vi "Special_Processing.vi"(6 "cluster in":T1, 8 "error in (no error)":errorcluster, 9 "Terminal Map In":map{string, T3}(c390), 10 "Wires":T2[](array[typedef]), 11 "GrowableObjectFunction in":refnum<class "PropertyNode.lvclass">) -> (0 "error out":errorcluster, 1 "Terminal Map Out":map{string, T3}(c390), 2 "Wires out":T2[](array[typedef]), 3 "GrowableObjectFunction out":refnum<class "PropertyNode.lvclass">)   [LabVIEW 2025, in "PropertyNode.lvclass"]
uses:
  PropertyNode.lvclass
  C:/Users/mrjak/Documents/GitHub/LVGPT/LabVIEW/VIs/Classes/Node/Node.lvclass
  Controls/wire.ctl
  Controls/Terminal.ctl
  Controls/bd.ctl
  Node.lvclass
  Node.lvclass/Node.ctl
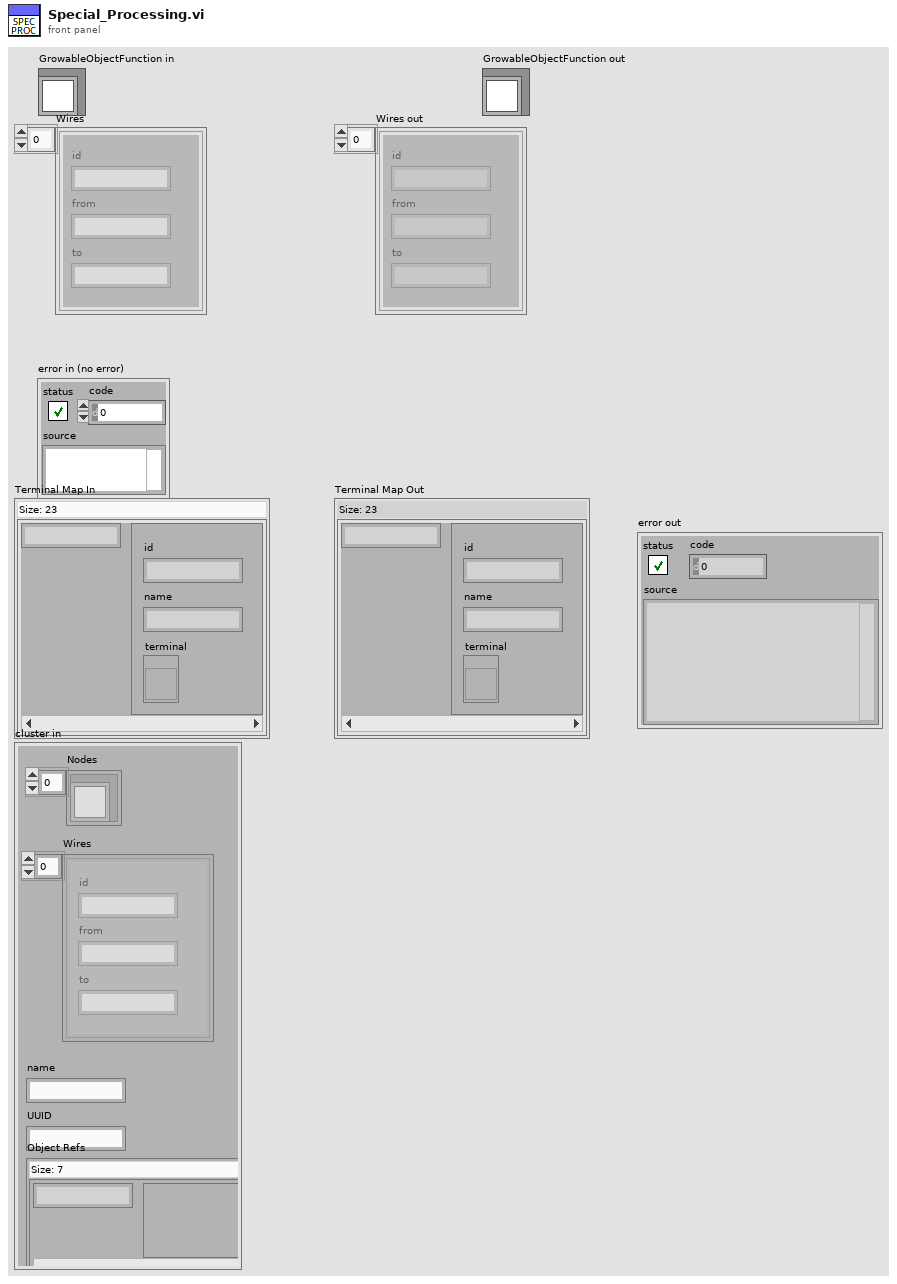
[diagram p1: front panel]
types:
  T1 = typedef "bd.ctl" = cluster{"Nodes":refnum<class "Node.lvclass">[], "Wires":T2[], "name":string, "UUID":string, "Object Refs":map{string, variant}}
  T2 = typedef "wire.ctl" = cluster{"id":string, "from":string, "to":string}
  T3 = typedef "Terminal.ctl" = cluster{"id":string, "name":string, "terminal":refnum<vi>}
  T4 = typedef "GrowableFunctionNode.ctl" = cluster{"terminalUUID":string, "Write":bool}
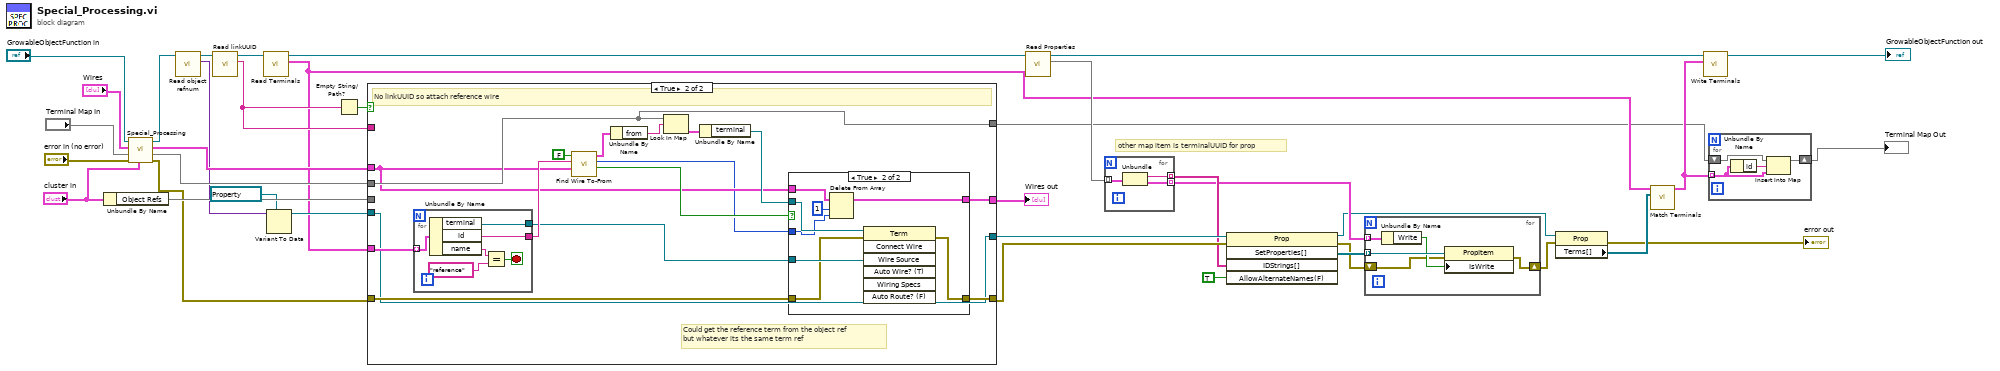
[diagram p0: block diagram]
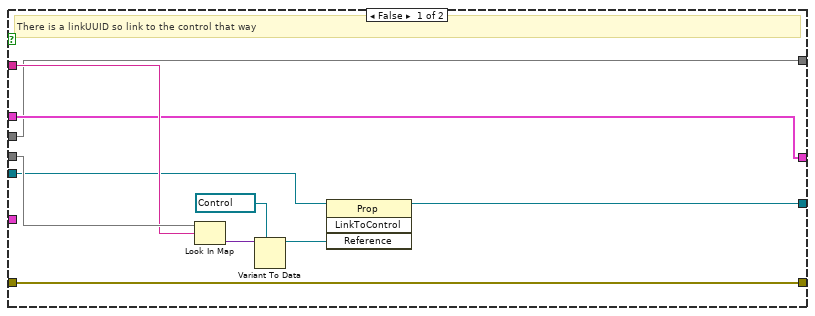
[diagram p2: hidden frame]
diagram:
  # "other map item is terminalUUID for prop"
  n1 = Unbundle By Name("cluster in") -> ("Object Refs"=w29:map{string, variant})
  n2 = call-parent "Special_Processing.vi"("cluster in"="cluster in", "error in (no error)"="error in (no error)", "Terminal Map In"="Terminal Map In", "Wires"="Wires", "Node in"="GrowableObjectFunction in") -> ("error out"=w22:errorcluster, "Terminal Map Out"=w23:map{string, T3}, "Wires out"=w26:T2[], "Node out"=w37:refnum<class "PropertyNode.lvclass">)  [unwired: 3 in]
  n3 = call-dynamic "Read object refnum.vi"("Node in"=w37) -> ("object refnum"=w18:variant, "Node out"=w32:refnum<class "PropertyNode.lvclass">)  [unwired: 8 in, 1 out]
  n4 = call-dynamic "Read linkUUID.vi"("GrowableObjectFunction in"=w32) -> ("linkUUID"=w28:string, "GrowableObjectFunction out"=w31:refnum<class "PropertyNode.lvclass">)  [unwired: 8 in, 1 out]
  n5 = call "Read Terminals.vi"("Node in"=w31) -> ("Terminals"=w12:T3[], "Node out"=w25:refnum<class "PropertyNode.lvclass">)  [unwired: 8 in, 1 out]
  n6 = Variant To Data(type=refnum<vi> refnum ("reference"), Variant=w18) -> (data=w19:refnum<vi>)  [unwired: 1 in, 1 out]
  n7 = Empty String/Path?(string/path=w28) -> (empty?=w30:bool)
  n8 = case shown="True" w30 {
    tunnel: w29 -> [w47 _]
    tunnel: w28 -> [w46 _]
    tunnel: w26 -> [w42 w50]
    tunnel: w12 -> [_ w63]
    tunnel: [w42 w48] -> w24
    tunnel: w23 -> [w40 w53]
    tunnel: w22 -> [w41 w55]
    tunnel: [w41 w54] -> w16
    tunnel: [w40 w53] -> w7
    tunnel: w19 -> [w39 w52]
    tunnel: [w38 w52] -> w17
    frame False {
      # "There is a linkUUID so link to the control that way"
      n9 = Look In Map(map=w47, key=w46) -> (value=w45:variant)  [unwired: 1 in, 1 out]
      n10 = Variant To Data(type=refnum<vi> refnum ("Reference"), Variant=w45) -> (data=w43:refnum<vi>)  [unwired: 1 in, 1 out]
      n11 = invoke class="Prop" method="LinkToControl"(reference=w39, "Reference"=w43) -> (reference out=w38:refnum<vi>)  [unwired: 2 in, 3 out]
    }
    frame True {
      # "Could get the reference term from the object ref \nbut whatever its the same term ref"
      # "No linkUUID so attach reference wire"
      n12 = for {
        tunnel: w63 -> [w79] mode=indexing
        tunnel: [w75] -> w62
        tunnel: [w74] -> w56
        stop <- w76 stop-if-true
        n13 = Unbundle By Name(w79) -> ("terminal"=w74:refnum<vi>, "id"=w75:string, "name"=w78:string)
        n14 = Equal?(x=w78, y="reference") -> (x = y?=w76:bool)
      }
      n15 = call "Find Wire To-From.vi"("Wires"=w50, "termUUID"=w62, "From UUID?"=FALSE) -> ("Found"=w51:bool, "Index"=w49:i32, "Wire"=w60:T2)  [unwired: 6 in]
      n16 = Unbundle By Name(w60) -> ("from"=w59:string)
      n17 = Look In Map(map=w53, key=w59) -> (value=w58:T3)  [unwired: 1 in, 1 out]
      n18 = Unbundle By Name(w58) -> ("terminal"=w57:refnum<vi>)
      n19 = case shown="True" w51 {
        tunnel: w57 -> [_ w73]
        tunnel: w56 -> [_ w72]
        tunnel: w55 -> [w65 w71]
        tunnel: [w65 w70] -> w54
        tunnel: w50 -> [w64 w69]
        tunnel: w49 -> [_ w67]
        tunnel: [w64 w66] -> w48
        frame False {
        }
        frame True {
          n20 = Delete From Array(array=w69, length=1, index=w67) -> (array with subset deleted=w66:T2[])  [unwired: 1 out]
          n21 = invoke class="Term" method="Connect Wire"(reference=w73, error in=w71, "Wire Source"=w72) -> (error out=w70:errorcluster)  [unwired: 4 in, 6 out]
        }
      }
    }
  }
  "Wires out" <- w24
  n22 = call-dynamic "Read Properties.vi"("PropertyNode in"=w25) -> ("Properties"=w15:map{string, T4}, "PropertyNode out"=w21:refnum<class "PropertyNode.lvclass">)  [unwired: 8 in, 1 out]
  n23 = for {
    tunnel: w15 -> [w82] mode=indexing
    tunnel: [w81] -> w14 mode=indexing
    tunnel: [w80] -> w4 mode=indexing
    n24 = Unbundle(w82) -> (w81:string, "GrowableFunctionNode"=w80:T4)
  }
  n25 = invoke class="Prop" method="SetProperties[]"(reference=w17, error in=w16, "IDStrings[]"=w14, "AllowAlternateNames(F)"=TRUE ("Allow Alternate Names? (F)")) -> (reference out=w3:refnum<vi>, error out=w2:errorcluster, "SetProperties[]"=w5:refnum<vi>[])  [unwired: 1 in, 2 out]
  n26 = for {
    tunnel: w5 -> [w87] mode=indexing
    tunnel: w4 -> [w86] mode=indexing
    shift-right: [w83] -> w1
    shift-left: w2 -> [w84]
    n27 = Unbundle By Name(w86) -> ("Write"=w85:bool)
    n28 = property class="PropItem"(reference=w87, error in=w84, "IsWrite"=w85) -> (error out=w83:errorcluster)  [unwired: 1 out]
  }
  n29 = property class="Prop"(reference=w3, error in=w1) -> (error out=→"error out":errorcluster, "Terms[]"=w11:refnum<vi>[])  [unwired: 1 out]
  n30 = call "Match Terminals.vi"("Terms[]"=w11, "Terminals"=w12) -> ("Terminals Out"=w8:T3[])  [unwired: 9 in]
  n31 = call "Write Terminals.vi"("Terminals"=w8, "Node in"=w21) -> ("Node out"=→"GrowableObjectFunction out":refnum<class "PropertyNode.lvclass">)  [unwired: 8 in, 1 out]
  n32 = for {
    shift-right: [w90] -> w6
    shift-left: w7 -> [w91]
    tunnel: w8 -> [w89] mode=indexing
    n33 = Unbundle By Name(w89) -> ("id"=w88:string)
    n34 = Insert Into Map(map in=w91, key=w88, value=w89) -> (map out=w90:map{string, T3})  [unwired: 2 out]
  }
  "Terminal Map Out" <- w6
